vi "YPRGlobal.vi"(0 "Yaw":dbl, 1 "Pitch":dbl, 2 "Roll":dbl, 3 "Compass Heading":dbl, 7 "Byte Count":u32, 8 "Update":bool, 10 "Initialize":bool) -> (20 "Yaw Out":dbl, 21 "Pitch Out":dbl, 22 "Roll Out":dbl, 23 "Compass Heading Out":dbl, 25 "Last Update":dbl, 26 "Update Count":i32, 27 "Byte Count Out":u32)   [LabVIEW 2015, in "Nav6.lvlib"]
uses:
  Nav6.lvlib
  <vilib>/Rock Robotics/SystemInterfaces/Utilities/FPGA_UtilitiesRead LocalTime.vi
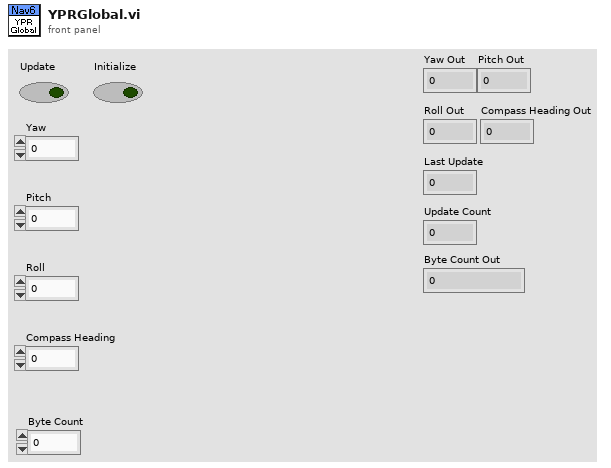
[diagram p1: front panel]
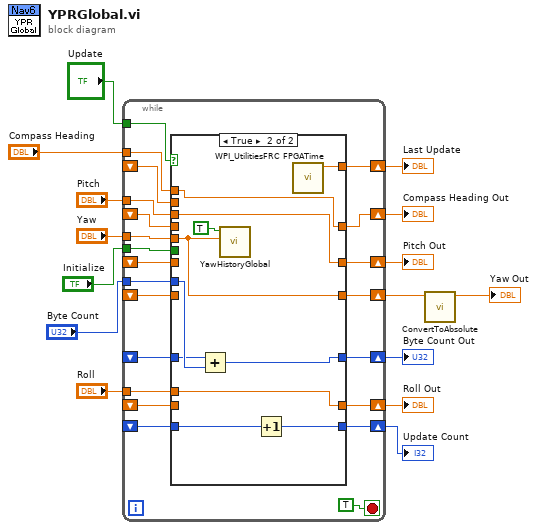
[diagram p0: block diagram]
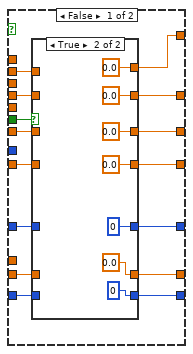
[diagram p2: hidden frame]
diagram:
  n1 = while {
    shift-right: [w35] -> w1
    shift-left: _ -> [w28]
    shift-right: [w33] -> w11
    shift-left: _ -> [w27]
    shift-right: [w31] -> w10
    shift-left: _ -> [w26]
    shift-right: [w29] -> w9
    shift-left: _ -> [w25]
    tunnel: "Yaw" -> [w36]
    tunnel: "Pitch" -> [w34]
    tunnel: "Roll" -> [w32]
    tunnel: "Compass Heading" -> [w30]
    shift-right: [w24] -> w8
    shift-left: _ -> [w23]
    shift-right: [w22] -> w6
    shift-left: _ -> [w21]
    shift-right: [w19] -> w5
    shift-left: _ -> [w20]
    tunnel: "Byte Count" -> [w18]
    tunnel: "Update" -> [w17]
    tunnel: "Initialize" -> [w16]
    stop <- TRUE stop-if-true
    n2 = case shown="True" w17 {
      tunnel: [w51 w73] -> w35
      tunnel: w36 -> [_ w73]
      tunnel: [w49 w77] -> w33
      tunnel: w34 -> [_ w77]
      tunnel: [w47 w76] -> w31
      tunnel: w32 -> [_ w76]
      tunnel: [w45 w75] -> w29
      tunnel: w30 -> [_ w75]
      tunnel: w28 -> [w52 _]
      tunnel: w27 -> [w50 _]
      tunnel: w26 -> [w48 _]
      tunnel: w25 -> [w46 _]
      tunnel: [w43 w74] -> w24
      tunnel: w23 -> [w44 _]
      tunnel: [w41 w68] -> w22
      tunnel: w21 -> [w42 w67]
      tunnel: [w39 w69] -> w19
      tunnel: w20 -> [w40 w70]
      tunnel: w18 -> [_ w71]
      tunnel: w16 -> [w38 _]
      frame False {
        n3 = case shown="True" w38 {
          tunnel: w52 -> [w59 _]
          tunnel: [w59 0.0 ("Yaw")] -> w51
          tunnel: w50 -> [w58 _]
          tunnel: [w58 0.0 ("Pitch")] -> w49
          tunnel: w48 -> [w57 _]
          tunnel: [w57 0.0 ("Roll")] -> w47
          tunnel: w46 -> [w56 _]
          tunnel: [w56 0.0 ("Compass Heading")] -> w45
          tunnel: w44 -> [w55 _]
          tunnel: [w55 0.0 ("FPGA Time")] -> w43
          tunnel: w42 -> [w54 _]
          tunnel: [w54 u32 0] -> w41
          tunnel: w40 -> [w53 _]
          tunnel: [w53 u32 0] -> w39
          frame False {
          }
          frame True {
          }
        }
      }
      frame True {
        n4 = Add(x=w70, y=w71) -> (x+y=w69:u32)
        n5 = call "YawHistoryGlobal.vi"("Yaw"=w73, "Update"=TRUE) -> ()  [unwired: 9 in, 1 out]
        n6 = Increment(x=w67) -> (x+1=w68:u32)
        n7 = call <vilib>:"WPI_UtilitiesFRC FPGATime.vi"() -> ("FPGA Time"=w74:dbl)  [unwired: 10 in, 1 out]
      }
    }
  }
  "Pitch Out" <- w11
  "Roll Out" <- w10
  "Compass Heading Out" <- w9
  "Last Update" <- w8
  "Update Count" <- w6
  "Byte Count Out" <- w5
  n8 = call "ConvertToAbsolute.vi"("Yaw"=w1) -> ("Absolute Yaw"=→"Yaw Out":dbl)  [unwired: 10 in]
